vi "PRBS_bit_generator_indexer.vi"(10 "MLS array index\n\nNote: start from 0":i32, 11 "Bit Length\n(how many bits does the sequence have)":i64) -> (2 "mls sequence":u8[](array[numeric]), 3 "Numeric":u8)   [LabVIEW 2020]
uses:
  <vilib>/Simulation/Implementation/Shared/SIMSCR Execution Mode.ctl
  <vilib>/Simulation/Scripting/Companion Diagram/SimConfigNode/SimParams.ctl
  <vilib>/Simulation/Scripting/Companion Diagram/SimConfigNode/_simSolvers.ctl
  <vilib>/Simulation/Param Hierarchy/Typedefs/SIMPH Param Control Actions.ctl
  <vilib>/Simulation/Implementation/Shared/NILVSim_ParamChanged.vi
  <vilib>/Simulation/Implementation/Shared/NILVSIM_BeginStep.vi
  <vilib>/Simulation/Utility/Implementation/NILVSim Memory.llb/NILVSim Memory (core).vi
  <vilib>/Simulation/Implementation/Shared/SIM Is Init or Final Stage.vi
  <vilib>/Simulation/Implementation/Shared/NILVSim_Manager.vi
  <vilib>/Utility/error.llb/Clear Errors.vi
  <vilib>/Simulation/Implementation/Shared/NILVSim_FinalizeModel.vi
  <vilib>/Simulation/Implementation/Shared/SIM Unbundle Sim Info.vi
  <vilib>/Simulation/Implementation/Shared/NILVSim_Initialize.vi
  <vilib>/Simulation/Utility/Implementation/NILVSim Get Time and IsAcceptedStep.vi
  <vilib>/Simulation/Implementation/Shared/NILVSim_GetModelError.vi
  <vilib>/Simulation/Implementation/Shared/SIM SimErrorHandler.vi
  <vilib>/Simulation/Implementation/Shared/SIMSH Read Queue.vi
  <vilib>/Simulation/Implementation/Shared/SIM Bundle Sim Info.vi
  <vilib>/Simulation/Scripting/Companion Diagram/SimConfigNode/SimDog.xnode
  <vilib>/Analysis/NI_AALBase.lvlib
  <vilib>/Simulation/Implementation/XNodeFramework/SimXNode/SimX.xnode
  <vilib>/Simulation/Implementation/Shared/NI_SIM_Implementation.lvlib
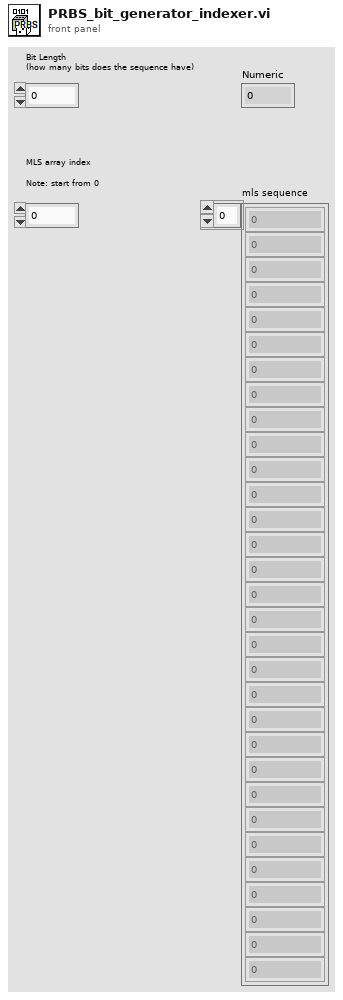
[diagram p1: front panel]
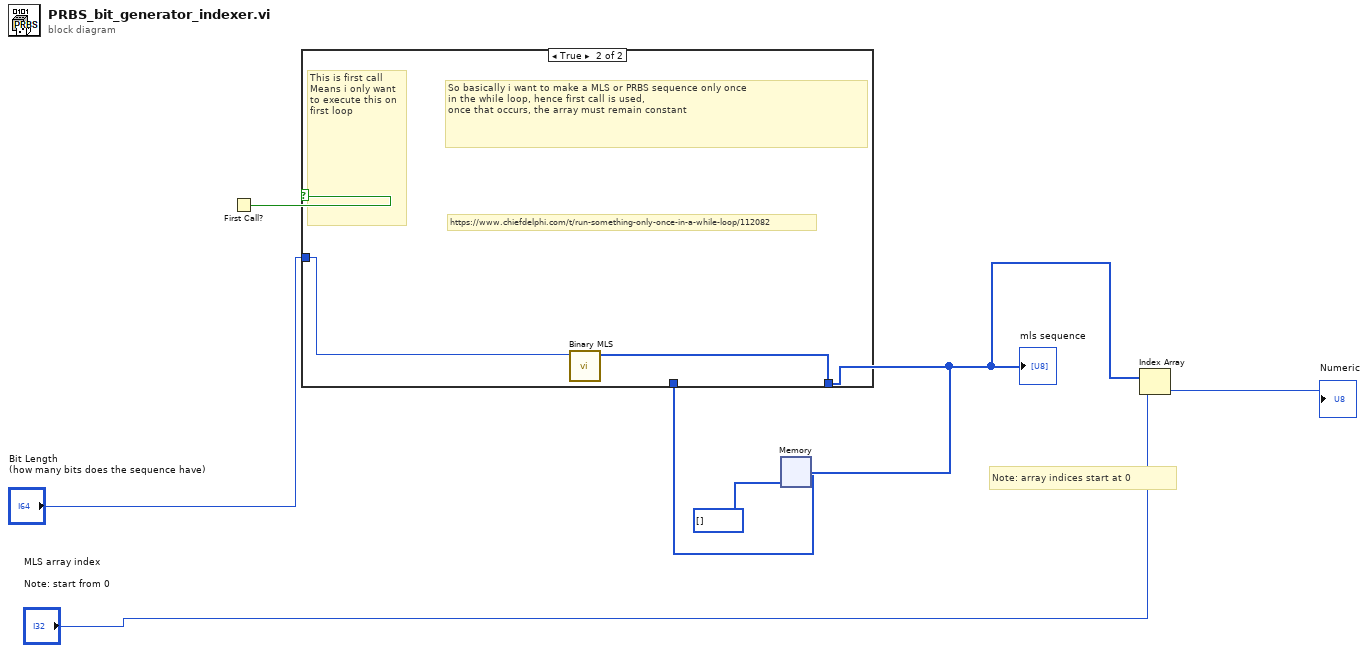
[diagram p0: block diagram]
diagram:
  # "Note: array indices start at 0"
  n1 = First Call?() -> (First Call?: T/F=w1:bool)
  n2 = case shown="True" w1 {
    tunnel: [w8 w10] -> w5
    tunnel: w2 -> [w8 _]
    tunnel: "Bit Length\n(how many bits does the sequence have)" -> [_ w9]
    frame False {
    }
    frame True {
      # "This is first call\nMeans i only want to execute this on first loop"
      # "So basically i want to make a MLS or PRBS sequence only once \nin the while loop, hence first call is used,\nonce that occurs, the array must remain constant"
      # "https://www.chiefdelphi.com/t/run-something-only-once-in-a-while-loop/112082"
      n3 = call <vilib>:"Binary MLS.vi"("samples"=w9) -> ("mls sequence"=w10:u8[])  [unwired: 9 in, 1 out]
    }
  }
  "mls sequence" <- w5
  n4 = xnode "Memory"("input"=w5, "initial value"=u8[] []) -> ("output"=w2:u8[])  [unwired: 4 in]
  n5 = Index Array(array=w5, index="MLS array index\n\nNote: start from 0") -> (element=→"Numeric":u8)
